vi "refresh C2 frequency.vi"(8 "error in (no error)":errorcluster, 11 "Waveform in":refnum<class "Waveform.lvclass">) -> (0 "error out":errorcluster, 3 "Waveform out":refnum<class "Waveform.lvclass">)   [LabVIEW 2012, in "Waveform.lvclass"]
uses:
  Waveform.lvclass
  Waveform.lvclass/Waveform.ctl
  <resource>/objmgr/daqmx.rc
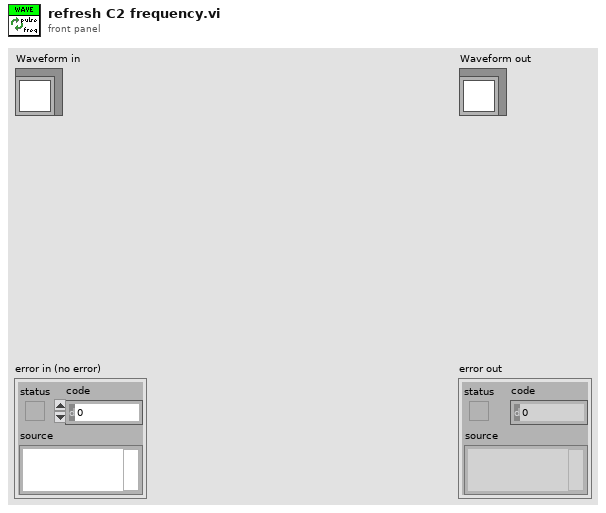
[diagram p1: front panel]
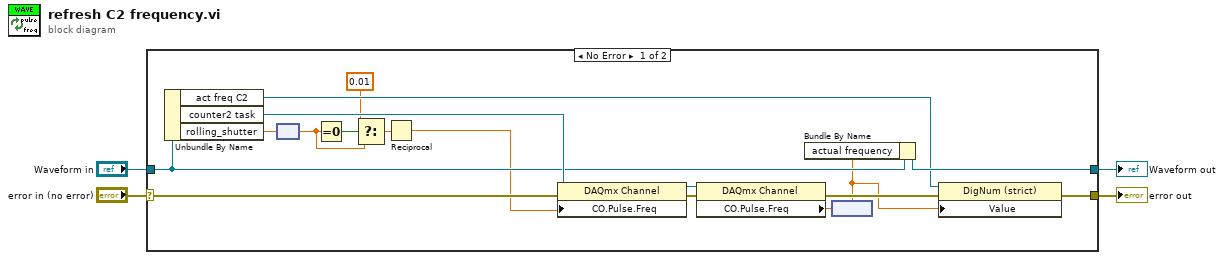
[diagram p0: block diagram]
diagram:
  n1 = case shown="No Error" "error in (no error)" {
    selector: "error in (no error)" -> [w15 w23]
    tunnel: [w13 w23] -> w3
    tunnel: [w17 w22] -> w1
    tunnel: "Waveform in" -> [w18 w22]
    frame No Error {
      n2 = Unbundle By Name(w18) -> ("act freq C2"=w12:refnum<vi>, "counter2 task"=w21:refnum<k21>, "rolling_shutter"=w10:dbl[unit])
      n3 = node(w10) -> (w8:dbl)
      n4 = Equal To 0?(x=w8) -> (x = 0?=w9:bool)
      n5 = Select(t=0.01, s=w9, f=w8) -> (s? t:f=w5:dbl)
      n6 = Reciprocal(x=w5) -> (1/x=w6:dbl)
      n7 = property class="DAQmx Channel"(reference=w21, error in=w15, "CO.Pulse.Freq"=w6) -> (reference out=w20:refnum<k21>, error out=w19:errorcluster)
      n8 = property class="DAQmx Channel"(reference=w20, error in=w19) -> (error out=w14:errorcluster, "CO.Pulse.Freq"=w16:dbl)  [unwired: 1 out]
      n9 = node(w16) -> (w11:dbl[unit])
      n10 = Bundle By Name(cluster=w18, "actual frequency"=w11) -> (w17:refnum<class "Waveform.lvclass">)
      n11 = property class="DigNum (strict)"(reference=w12, error in=w14, "Value"=w11) -> (error out=w13:errorcluster)  [unwired: 1 out]
    }
    frame Error {
    }
  }
  "error out" <- w3
  "Waveform out" <- w1
